vi "VA CoAP - Message - CREATE.vi"(7 "Message ID":u16, 8 "Token":string, 9 "Method Code":u8, 10 "Type":T1 items=["CONfimable", "NON-confirmable", "ACKnowledgement", "ReSeT"]) -> (2 "CoAP Message":string)   [LabVIEW 2020]
uses:
  data types/VA CoAP - Message - Type.ctl
panel:
  out "Token Lenght":bool[](array[boolean])
  out "Type":bool[](array[boolean])
  out "ORG Hex":u32 format="%x"
  out "ORG":i32 format="%08b"
  out "Hex":u32 format="%x"
  out "BIN":u32 format="%08b"
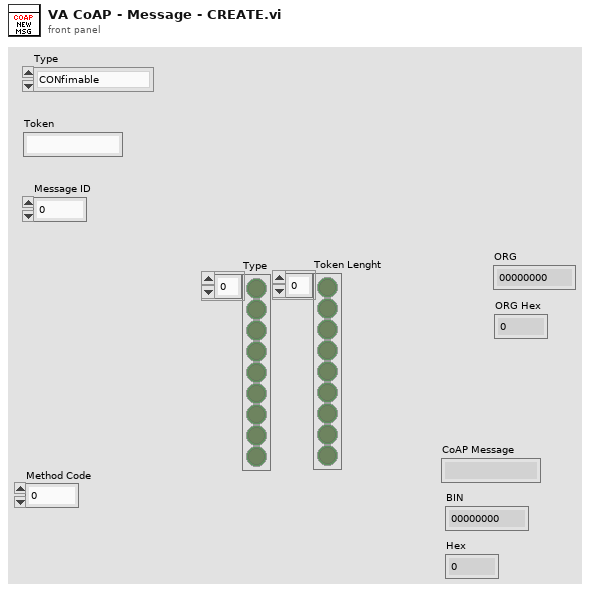
[diagram p1: front panel]
types:
  T1 = typedef "VA CoAP - Message - Type.ctl" = u8
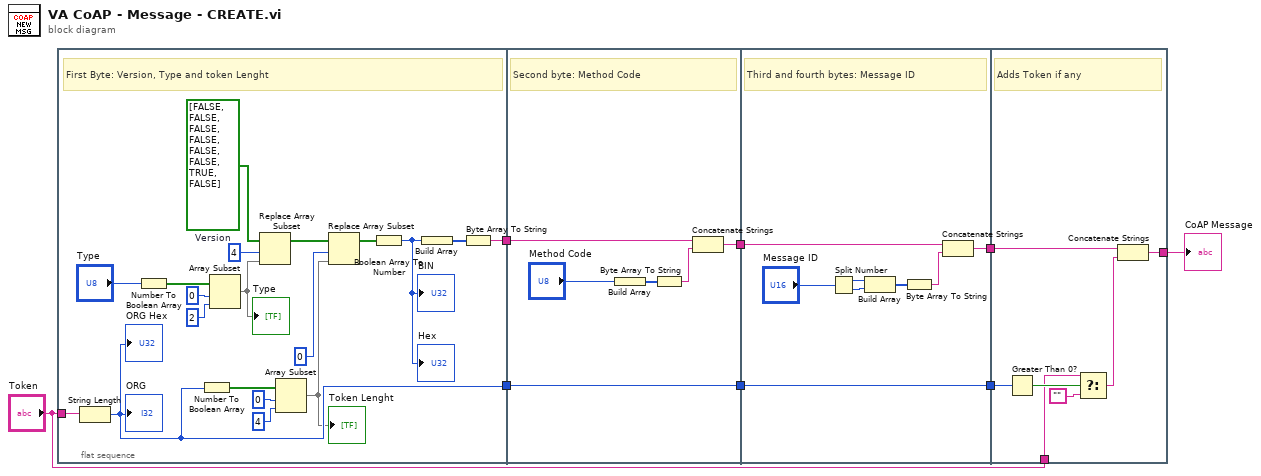
[diagram p0: block diagram]
diagram:
  n1 = flat-sequence {
    tunnel: "Token" -> [w27]
    tunnel: [w24] -> w8
    tunnel: [w23] -> w7
    tunnel: w8 -> [w29]
    tunnel: [w30] -> w6
    tunnel: w7 -> [w33]
    tunnel: [w33] -> w4
    tunnel: w6 -> [w36]
    tunnel: [w40] -> w5
    tunnel: w4 -> [w41]
    tunnel: [w41] -> w3
    tunnel: [w42] -> w2
    tunnel: w5 -> [w44]
    tunnel: w3 -> [w48]
    tunnel: "Token" -> [w46]
    frame #0 {
      w17 = bool[] [FALSE, FALSE, FALSE, FALSE, FALSE, FALSE, TRUE, FALSE]  # Version
      # "First Byte: Version, Type and token Lenght"
      n2 = String Length(string=w27) -> (length=w23:i32)
      "ORG" <- w23
      "ORG Hex" <- w23
      n3 = Number To Boolean Array(number="Type") -> (Boolean array=w18:bool[])
      n4 = Number To Boolean Array(number=w23) -> (Boolean array=w15:bool[])
      n5 = Array Subset(array=w18, index=0, length=2) -> (w20:bool[])
      "Type" <- w20
      n6 = Replace Array Subset(array=w17, new element=w20, index=4) -> (w16:bool[])
      n7 = Array Subset(array=w15, index=0, length=4) -> (w12:bool[])
      "Token Lenght" <- w12
      n8 = Replace Array Subset(array=w16, new element=w12, index=0) -> (w10:bool[])
      n9 = Boolean Array To Number(Boolean array=w10) -> (number=w26:u32)
      "BIN" <- w26
      "Hex" <- w26
      n10 = Build Array(w26) -> (w25:u32[])
      n11 = Byte Array To String(unsigned byte array=w25) -> (string=w24:string)
    }
    frame #1 {
      # "Second byte: Method Code"
      n12 = Build Array("Method Code") -> (w31:u8[])
      n13 = Byte Array To String(unsigned byte array=w31) -> (string=w28:string)
      n14 = Concatenate Strings(w29, w28) -> (w30:string)
    }
    frame #2 {
      # "Third and fourth bytes: Message ID"
      n15 = Split Number(x="Message ID") -> (hi(x)=w39:u8, lo(x)=w38:u8)
      n16 = Build Array(w39, w38) -> (w37:u8[])
      n17 = Byte Array To String(unsigned byte array=w37) -> (string=w35:string)
      n18 = Concatenate Strings(w36, w35) -> (w40:string)
    }
    frame #3 {
      # "Adds Token if any"
      n19 = Greater Than 0?(x=w48) -> (x > 0?=w47:bool)
      n20 = Select(t=w46, s=w47, f="") -> (s? t:f=w43:string)
      n21 = Concatenate Strings(w44, w43) -> (w42:string)
    }
  }
  "CoAP Message" <- w2
